vi "CaLabEventUnregister.vi"(8 "error in (no error)":errorcluster, 10 "Refnum":refnum<event-registration>, 11 "Event":refnum<user-event>) -> (0 "error out":errorcluster)   [LabVIEW 2020]
doc: "This is a VI for creating user events.\nINPUT:\n <b>PV Name</b>\n name of EPICS variable\n <b>Field Names</b>\n optional\n string array of EPICS fields (\"EGU\", \"DESCRIPTION\" etc.)\n <b>Timeout</b>\n optional\n timeout for Channel Access requests\n default value: 3 seconds\n <b>Error in (no error)</b>\n\nOUTPUT:\n <b>Event</b>\n event structure\n <b>Refnum</b>\n event registration number\n <b>Error out</b>"
uses:
  libcalab.so
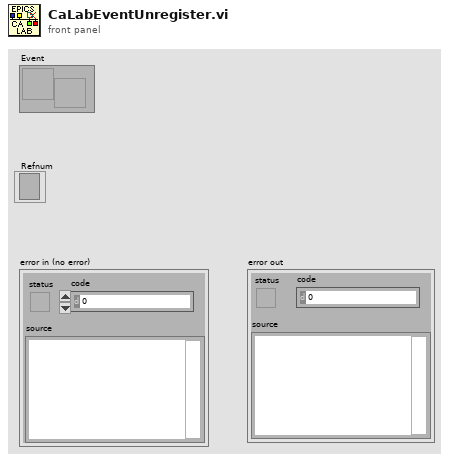
[diagram p1: front panel]
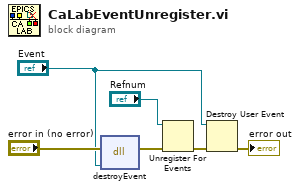
[diagram p0: block diagram]
diagram:
  n1 = dll-call lib="usr/local/calab/libcalab.so" fn="destroyEvent" label="add event"(error in="error in (no error)", "RefNum"="Event") -> (error out=w2:errorcluster)  [unwired: 2 in, 3 out]
  n2 = Unregister For Events(event registration refnum="Refnum", error in=w2) -> (error out=w1:errorcluster)
  n3 = Destroy User Event(user event="Event", error in=w1) -> (error out=→"error out":errorcluster)
